vi "hmi_swap_interface.vi"(8 "error in (no error)":errorcluster, 10 "interface":T1, 11 "subpanel_reference":refnum<vi>) -> (0 "error out":errorcluster)   [LabVIEW 2015, in "lv-interface-dom-nre.lvlib"]
uses:
  lv-interface-dom-nre.lvlib
  lv-interface-sub-common/_controls/interface_selection.ctl
  lv-interface-sub-common/lv-interface-sub-common.lvlib
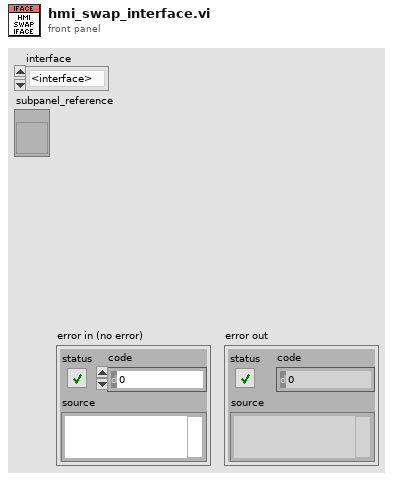
[diagram p1: front panel]
types:
  T1 = typedef "lv-interface-sub-common.lvlib/interface_selection.ctl" = enum16{"<interface>", "sub_interface_1", "sub_interface_2", "<null>"}
  T2 = typedef "lv-interface-dom-nre.lvlib/interface_refnum.ctl" = refnum<vi>
  T3 = enum32{"Invalid", "Standard", "Closed", "Hidden", "Minimized", "Maximized"}
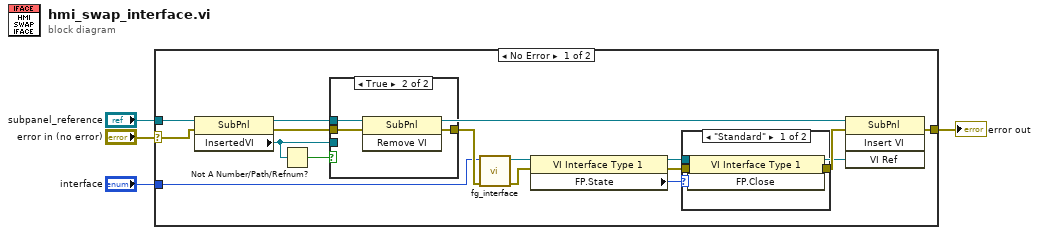
[diagram p0: block diagram]
diagram:
  n1 = case shown="No Error" "error in (no error)" {
    selector: "error in (no error)" -> [w17 w27]
    tunnel: "interface" -> [w13 _]
    tunnel: [w7 w27] -> w2
    tunnel: "subpanel_reference" -> [w5 _]
    frame No Error {
      n2 = property class="SubPnl"(reference=w5, error in=w17) -> (error out=w14:errorcluster, "InsertedVI"=w16:refnum<vi>)  [unwired: 1 out]
      n3 = Not A Number/Path/Refnum?(number/path/refnum=w16) -> (NaN/Path/Refnum?=w15:bool)
      n4 = case shown="True" w15 {
        tunnel: w16 -> [_ _]
        tunnel: w5 -> [_ w26]
        tunnel: w14 -> [w23 w25]
        tunnel: [w23 w24] -> w18
        frame False {
        }
        frame True {
          n5 = invoke class="SubPnl" method="Remove VI"(reference=w26, error in=w25) -> (error out=w24:errorcluster)  [unwired: 1 in, 2 out]
        }
      }
      n6 = call "fg_interface.vi"("error in (no error)"=w18, "interface"=w13) -> ("error out"=w12:errorcluster, "interface"=w6:T2)  [unwired: 7 in, 1 out]
      n7 = property class="VI Interface Type 1"(reference=w6, error in=w12) -> (reference out=w10:T2, error out=w9:errorcluster, "FP.State"=w11:T3)
      n8 = case shown="\"Standard\"" w11 {
        tunnel: w10 -> [w21 _]
        tunnel: w9 -> [w20 w22]
        tunnel: [w19 w22] -> w8
        frame "Standard" {
          n9 = invoke class="VI Interface Type 1" method="FP.Close"(reference=w21, error in=w20) -> (error out=w19:errorcluster)  [unwired: 1 in, 2 out]
        }
        frame Default {
        }
      }
      n10 = invoke class="SubPnl" method="Insert VI"(reference=w5, error in=w8, "VI Ref"=w6) -> (error out=w7:errorcluster)  [unwired: 1 in, 3 out]
    }
    frame Error {
    }
  }
  "error out" <- w2
